vi "DAQmx Create Channel (AI-Charge).vi"(0 "task in":refnum<k21>, 1 "maximum value":dbl=1e-09 format="%0.9f", 2 "minimum value":dbl=-1e-09 format="%0.9f", 3 "input terminal configuration":i32(ring)=-1 items=["Default"=-1, "RSE"=10083, "NRSE"=10078, "Differential"=10106, "Pseudodifferential"=12529], 5 "physical channels":tag, 7 "name to assign":string, 9 "units":i32(ring)=16102 items=["Coulombs"=16102, "pCoulombs"=16103, "From Custom Scale"=10065], 11 "error in":errorcluster, 12 "custom scale name":tag) -> (4 "task out":refnum<k21>, 15 "error out":errorcluster)   [LabVIEW 2013]
doc: "Creates channel(s) that use a sensor with charge output."
uses:
  nilvaiu.dll
panel:
  # "input limits"
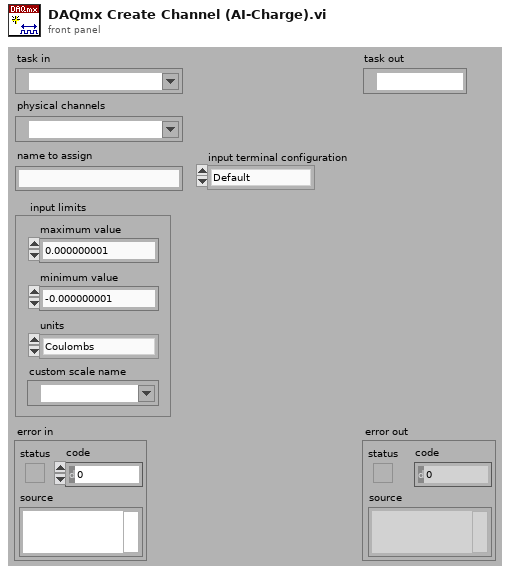
[diagram p1: front panel]
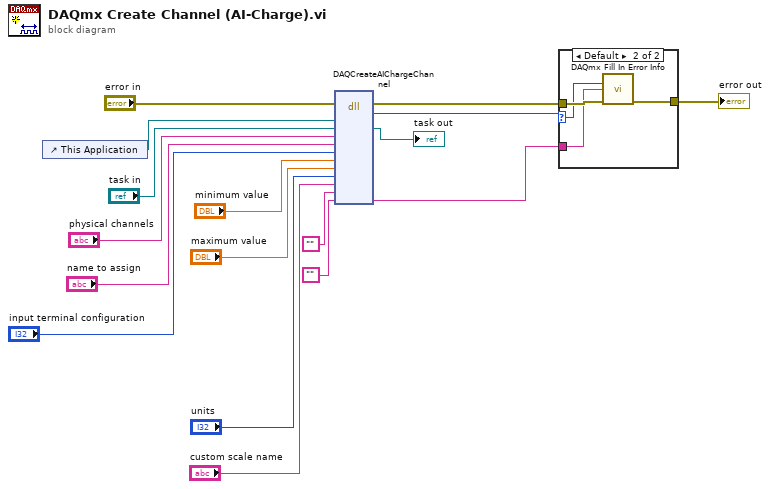
[diagram p0: block diagram]
diagram:
  n1 = control-ref of="This Application"() -> (w16:refnum<vi>)
  n2 = dll-call lib="nilvaiu.*" fn="DAQCreateAIChargeChannel"(error in="error in", "lvAppReference"=w16, "taskID"="task in", "physical channel name"="physical channels", "virtual channel name"="name to assign", "input terminal configuration"="input terminal configuration", "minimum value"="minimum value", "maximum value"="maximum value", "units"="units", "customScale"="custom scale name", "channelNamesOut"="", "extendedErrorIndo"="") -> (error out=w4:errorcluster, "return type"=w2:i32, "taskID"=→"task out":refnum<k21>, "extendedErrorIndo"=w3:string)  [unwired: 11 in, 1 out]
  n3 = case shown="Default" w2 {
    selector: w2 -> [_ w20]
    tunnel: w4 -> [w18 w22]
    tunnel: [w18 w21] -> w5
    tunnel: w3 -> [_ w19]
    frame 0 {
    }
    frame Default {
      n4 = call "DAQmx Fill In Error Info.vi"("status code"=w20, "extended error info"=w19, "error in"=w22) -> ("error out"=w21:errorcluster)  [unwired: 1 in, 11 out]
    }
  }
  "error out" <- w5
